vi "MotorUI.vi"() -> ()   [LabVIEW 2011]
uses:
  MotorPosType.ctl
  Typedefs/XYf.ctl
  MotorStateType.ctl
  Typedefs/CmdEnum_MotorIn.ctl
  MotorAxisEnum.ctl
  MotorCmd_MoveToLimit.ctl
  GlobalVariables.vi
panel:
  in  "Cam XY Control":T1
  out "Cam Y":sgl
  out "Cam X":sgl
  in  "Save config":bool
  in  "Piezo XY":T1
  out "Piezo Y":sgl
  out "Piezo X":sgl
  out "Focal depth (um):":sgl
  out "Rotation (turns):":sgl
  out "Position: (mm)":sgl
  out "Motor update lag counter":i32
  in  "Rotation speed\n(turns/s)":sgl=1.0
  in  "Magnet offset":sgl
  in  "Piezo step pageup/down":sgl=2.0
  in  "Magnet home":bool
  in  "Reset magnet zero pos":bool
  out "Offset":T2
  in  "MotorState (initial value)":T3
  in  "Step size of up/down buttons":sgl=3.0
  in  "Motors Initialized?":bool
  out "motor cmd queue len":i32
  out "Current Position":T2
  in  "Piezo position":sgl
  in  "Magnet position [mm]":sgl
  in  "Rotation [turns]":sgl
  in  "Move magnet up":bool
  in  "Move magnet down":bool
  in  "Magnet rotation: Alternate 0/10":bool
  in  "Piezo stage down":bool
  in  "Piezo stage up":bool
  in  "Piezo step:":sgl=5.0
  # "Magnet Z"
  # "Focal depth"
  # "Magnet Rotation"
  # "Piezo XY"
  # "Magnet position:\nThe shown 'magnet position' cannot go below zero, so you can use the offset to set a lower magnet limit (in order to protect your flowcell)"
  # "Camera XY"
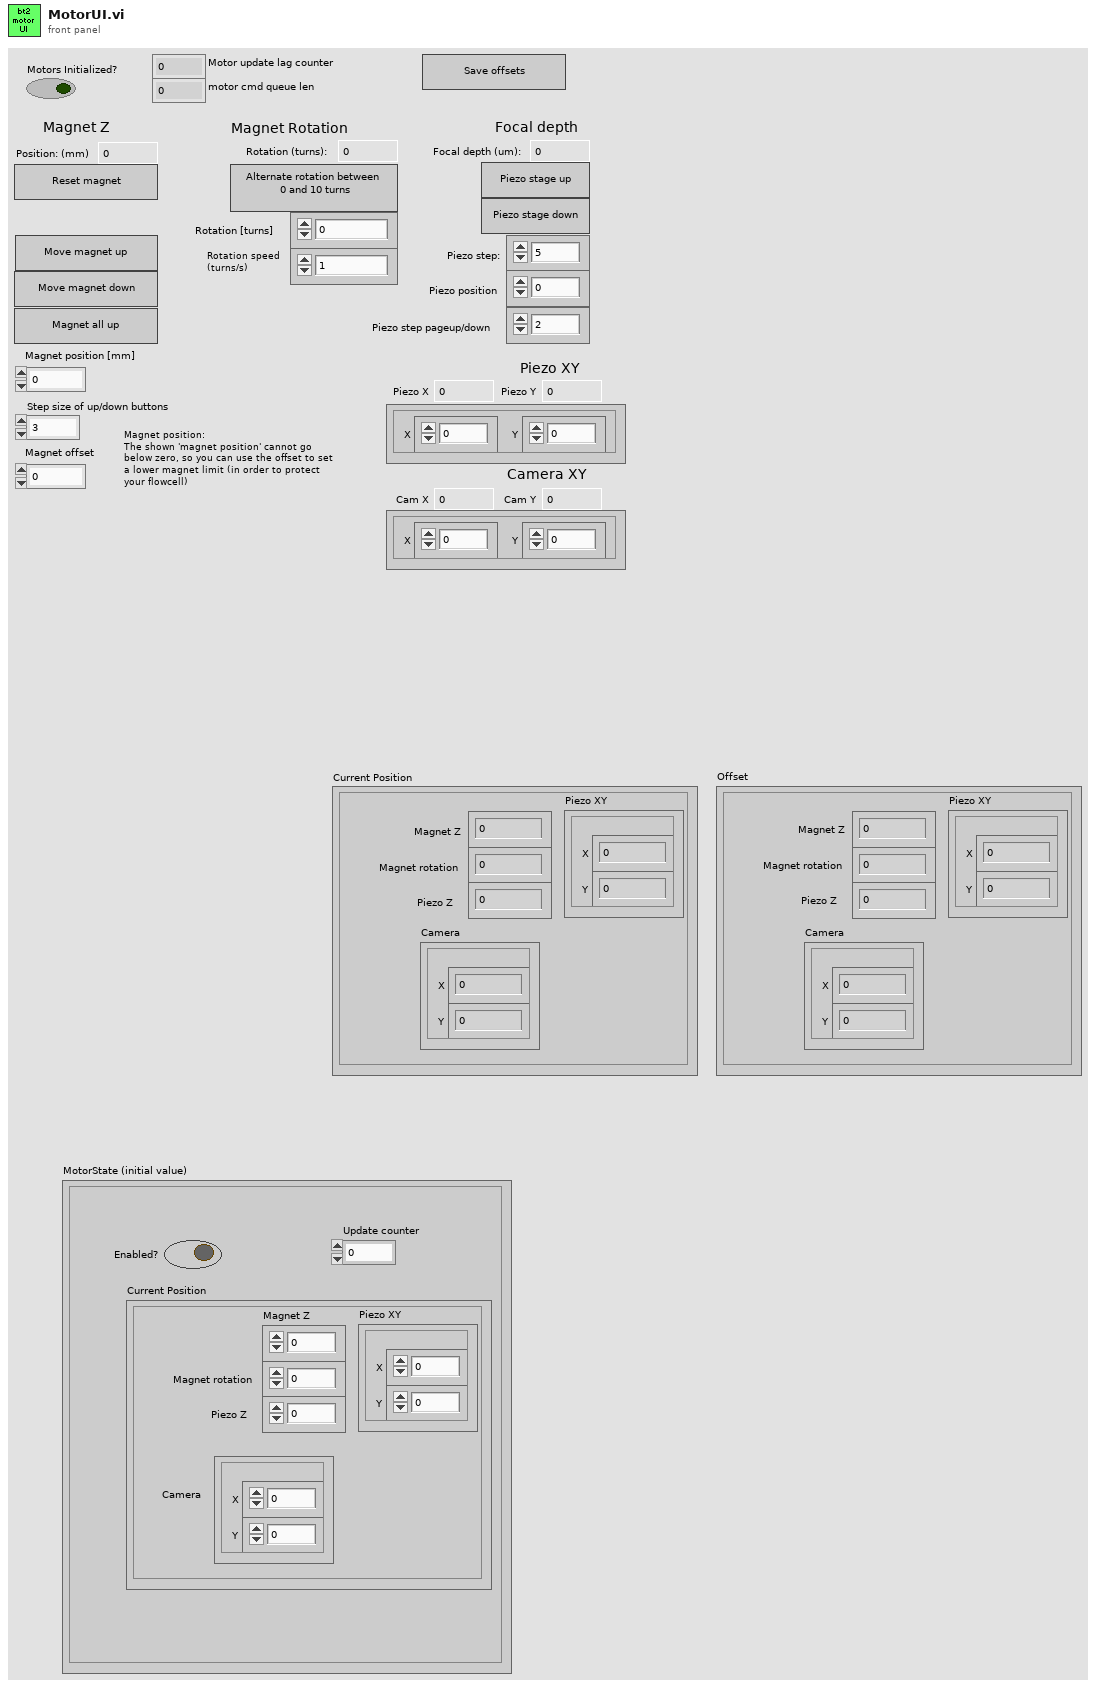
[diagram p1: front panel]
types:
  T1 = typedef "XYf.ctl" = cluster{"X":sgl, "Y":sgl}
  T2 = typedef "MotorPosType.ctl" = cluster{"Magnet Z":dbl, "Magnet rotation":dbl, "Camera":T1, "Piezo XY":T1, "Piezo Z":dbl}
  T3 = typedef "MotorStateType.ctl" = cluster{"Enabled?":bool, "Current Position":T2, "Update counter":i32}
  T4 = typedef "MotorConfigType.ctl" = cluster{"Offset":T2, "Maximum pos":T2, "Min limited?":T5, "Max limited?":T5, "Has velocity support":T5, "Default velocity":T2}
  T5 = typedef "MotorPosFlagsType.ctl" = cluster{"Magnet Z":bool, "Magnet rotation":bool, "Camera":cluster{"X":bool, "Y":bool}, "Piezo XY":cluster{"X":bool, "Y":bool}, "Piezo Z":bool}
  T6 = typedef "MotorAxisEnum.ctl" = enum16{"no axis", "magrot", "magpos", "px", "py", "pz", "camx", "camy"}
  T7 = typedef "CmdEnum_MotorIn.ctl" = enum32{"Init", "Close", "SetPosition", "UpdatePositions", "MoveToLimit"}
  T8 = typedef "MotorCmd_MoveToLimit.ctl" = cluster{"Motor Axis":T6, "Limit switch":enum16{"Positive", "Negative"}}
  T9 = typedef "eventvkey.ctl" = enum16{"ASCII", "Enter", "Return", "Shift", "Ctrl", "Alt", "Cmd", "Opt", "Caps", "NumLock", "Clear", "Break", "Up", "Down", "Left", "Right", "Insert", "Delete", "Home", "End", "PageUp", "PageDown", "Escape", "Help", "Pause", "ScrollLock", "F1", "F2", "F3", "F4", "F5", "F6", "F7", "F8", "F9", "F10", "F11", "F12", "F13", "F14", "F15", "F16", "F17", "F18", "F19", "F20", "F21", "F22", "F23", "F24", "Play", "VolumeUp", "VolumeDown", "Mute", "Two Byte Char"}
  T10 = typedef "QueueListType.ctl" = cluster{"Motor In":refnum<queue>, "User Interface Image View":refnum<queue>, "User Interface Camera Control":refnum<queue>, "User Interface Event Notifier":refnum<notifier>, "Initialized?":bool, "Experiment Script Event Notifier":refnum<notifier>}
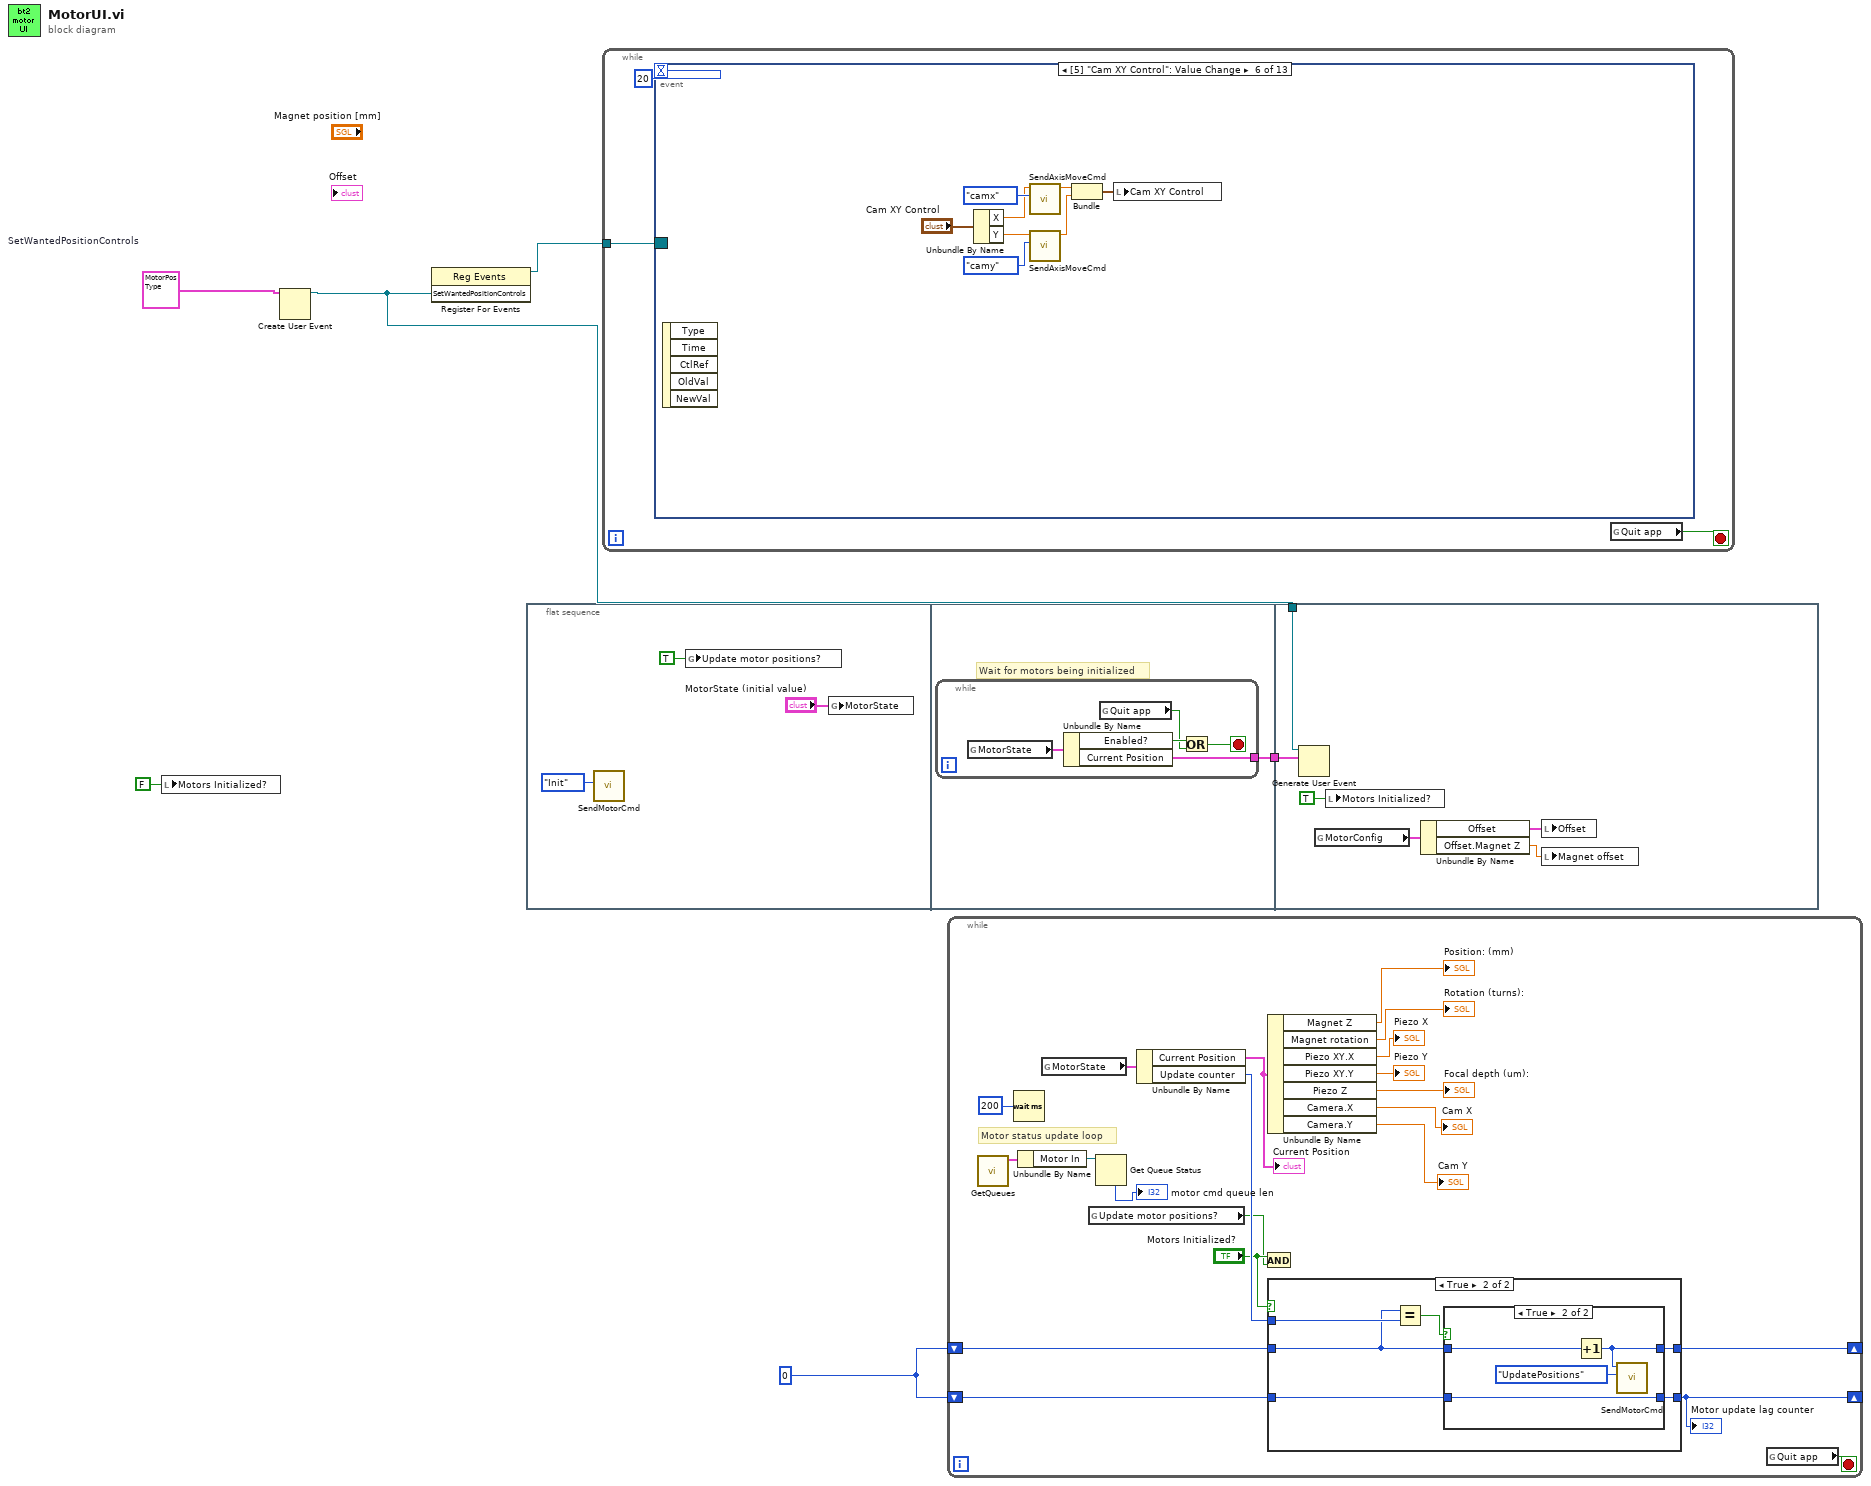
[diagram p0: block diagram]
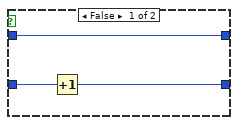
[diagram p3: hidden frame]
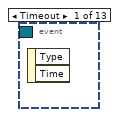
[diagram p4: hidden frame]
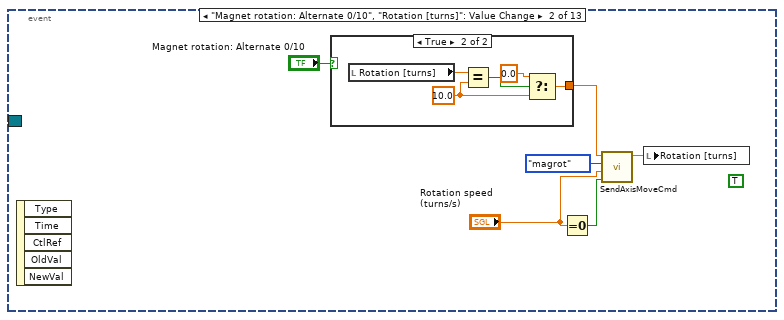
[diagram p5: hidden frame]
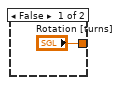
[diagram p6: hidden frame]
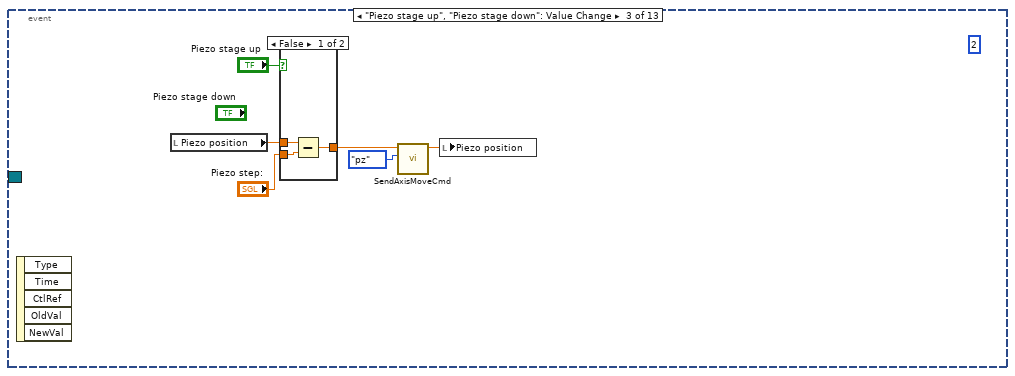
[diagram p7: hidden frame]
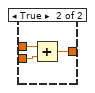
[diagram p8: hidden frame]
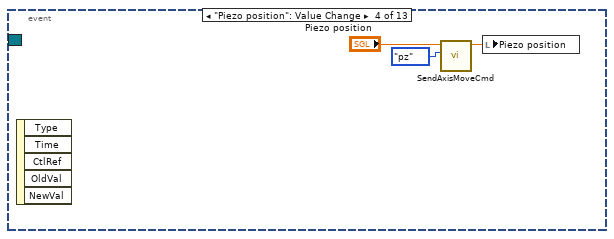
[diagram p9: hidden frame]
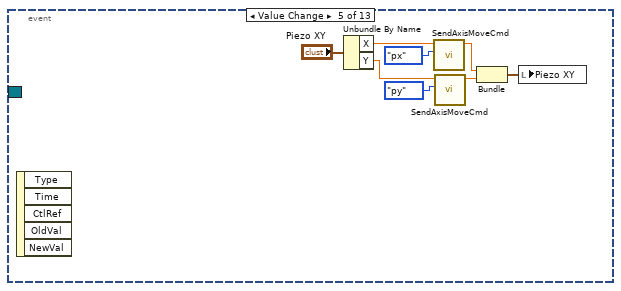
[diagram p10: hidden frame]
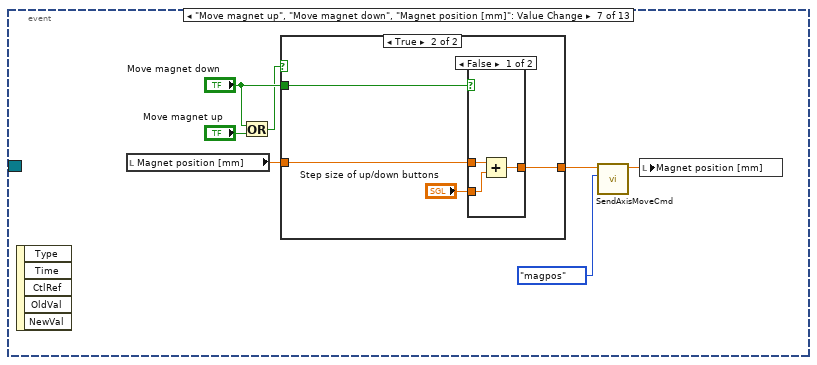
[diagram p11: hidden frame]
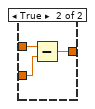
[diagram p13: hidden frame]
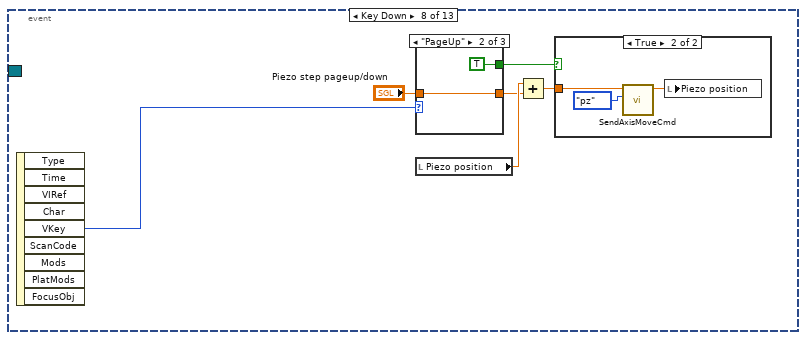
[diagram p14: hidden frame]
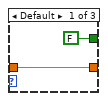
[diagram p16: hidden frame]
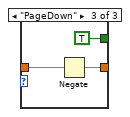
[diagram p17: hidden frame]
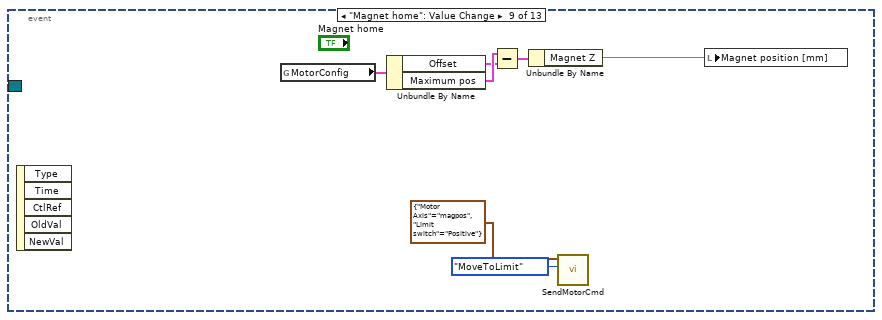
[diagram p18: hidden frame]
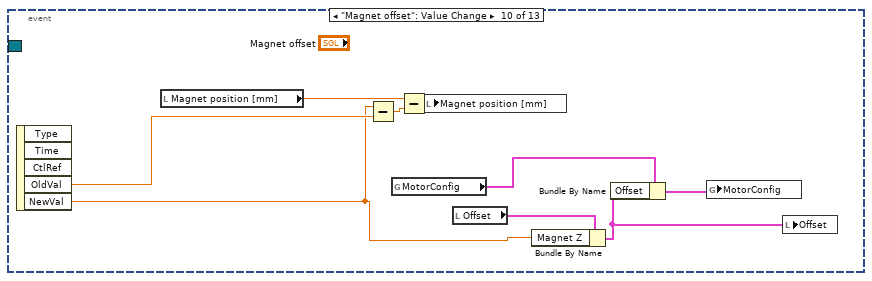
[diagram p19: hidden frame]
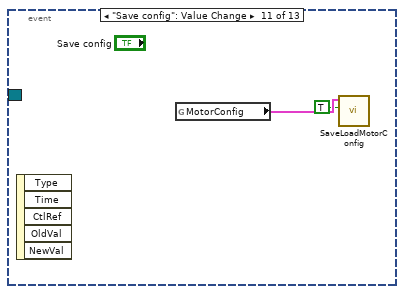
[diagram p20: hidden frame]
diagram:
  w4 = 0 ("Update counter")
  w5 = T2 {"Magnet Z"=0.0, "Magnet rotation"=0.0, "Camera"={"X"=0.0, "Y"=0.0}, "Piezo XY"={"X"=0.0, "Y"=0.0}, "Piezo Z"=0.0}  # SetWantedPositionControls
  n1 = local write "Motors Initialized?"(FALSE ("Motor Initialized?")) -> ()
  n2 = Create User Event(user event datatype=w5) -> (user event=w1:refnum<user-event>)  [unwired: 1 in, 1 out]
  n3 = register-events(w1) -> (reference out=w3:refnum<event-registration>)  [unwired: 2 in, 1 out]
  n4 = flat-sequence {
    tunnel: [w10] -> w2
    tunnel: w1 -> [w20]
    tunnel: w2 -> [w19]
    frame #0 {
      n5 = call "SendMotorCmd.vi"("Command Type"=enum16{"Init", "Close", "SetPosition"}."Init") -> ()  [unwired: 11 in]
      n6 = global write "GlobalVariables.vi" "Update motor positions?"(TRUE ("Update motor positions?")) -> ()
      n7 = global write "GlobalVariables.vi" "MotorState"("MotorState (initial value)") -> ()
    }
    frame #1 {
      # "Wait for motors being initialized"
      n8 = while {
        tunnel: [w14] -> w10
        stop <- w11 stop-if-true
        n9 = global read "GlobalVariables.vi" "MotorState"() -> (w15:T3)
        n10 = Unbundle By Name(w15) -> ("Enabled?"=w13:bool, "Current Position"=w14:T2)
        n11 = global read "GlobalVariables.vi" "Quit app"() -> (w12:bool)
        n12 = Or(x=w13, y=w12) -> (x .or. y?=w11:bool)
      }
    }
    frame #2 {
      n13 = Generate User Event(user event=w20, event data cluster=w19) -> ()  [unwired: 1 in, 2 out]
      n14 = global read "GlobalVariables.vi" "MotorConfig"() -> (w18:T4)
      n15 = local write "Motors Initialized?"(TRUE ("Motor Initialized?")) -> ()
      n16 = Unbundle By Name(w18) -> ("Offset"=w16:T2, "Offset.Magnet Z"=w17:dbl)
      n17 = local write "Offset"(w16) -> ()
      n18 = local write "Magnet offset"(w17) -> ()
    }
  }
  n19 = while {
    tunnel: w3 -> [w22]
    stop <- w23 stop-if-true
    n20 = event shown="[5] \"Cam XY Control\": Value Change" {
      selector: w22 -> [_ _ _ _ _ _ _ _ _ _ _ _ _]
      dyn-events: _ -> [_ _ _ _ _ _ _ _ _ _ _ _ _]
      timeout: 20 -> [_ _ _ _ _ _ _ _ _ _ _ _ _]
      event Timeout {
        n21 = event-data() -> ()  [unwired: 1 in, 2 out]
      }
      event "Magnet rotation: Alternate 0/10", "Rotation [turns]": Value Change {
        (unwired) TRUE ("Move flags.Magnet rotation")
        n22 = event-data() -> ()  [unwired: 1 in, 5 out]
        n23 = case shown="True" "Magnet rotation: Alternate 0/10" {
          tunnel: ["Rotation [turns]" w32] -> w28
          frame False {
          }
          frame True {
            w33 = sgl 10.0 ("y")
            n24 = local read "Rotation [turns]"() -> (w36:sgl)
            n25 = Equal?(x=w36, y=w33) -> (x = y?=w35:bool)
            n26 = Select(t=0.0, s=w35, f=w33) -> (s? t:f=w32:dbl)
          }
        }
        n27 = Equal To 0?(x="Rotation speed\n(turns/s)") -> (x = 0?=w25:bool)
        n28 = call "SendAxisMoveCmd.vi"("Instant? (T)"=w25, "Speed"="Rotation speed\n(turns/s)", "axis"=MotorAxisEnum."magrot", "Position"=w28) -> ("Limited pos"=w29:dbl)  [unwired: 7 in]
        n29 = local write "Rotation [turns]"(w29) -> ()
      }
      event "Piezo stage up", "Piezo stage down": Value Change {
        (unwired) 2 ("axis index")
        n30 = event-data() -> ()  [unwired: 1 in, 5 out]
        n31 = local read "Piezo position"() -> (w40:sgl)
        n32 = case shown="False" "Piezo stage up" {
          tunnel: w40 -> [w45 w48]
          tunnel: "Piezo step:" -> [w44 w47]
          tunnel: [w43 w46] -> w38
          frame False {
            n33 = Subtract(x=w45, y=w44) -> (x-y=w43:sgl)
          }
          frame True {
            n34 = Add(x=w48, y=w47) -> (x+y=w46:sgl)
          }
        }
        n35 = call "SendAxisMoveCmd.vi"("axis"=MotorAxisEnum."pz", "Position"=w38) -> ("Limited pos"=w39:dbl)  [unwired: 9 in]
        n36 = local write "Piezo position"(w39) -> ()
      }
      event "Piezo position": Value Change {
        n37 = event-data() -> ()  [unwired: 1 in, 5 out]
        n38 = call "SendAxisMoveCmd.vi"("axis"=MotorAxisEnum."pz", "Position"="Piezo position") -> ("Limited pos"=w49:dbl)  [unwired: 9 in]
        n39 = local write "Piezo position"(w49) -> ()
      }
      event Value Change {
        n40 = event-data() -> ()  [unwired: 1 in, 5 out]
        n41 = Unbundle By Name("Piezo XY") -> ("X"=w58:sgl, "Y"=w57:sgl)
        n42 = call "SendAxisMoveCmd.vi"("axis"=MotorAxisEnum."px", "Position"=w58) -> ("Limited pos"=w54:dbl)  [unwired: 9 in]
        n43 = call "SendAxisMoveCmd.vi"("axis"=MotorAxisEnum."py", "Position"=w57) -> ("Limited pos"=w53:dbl)  [unwired: 9 in]
        n44 = Bundle("Limited pos"=w54, "Limited pos"=w53) -> (w52:cluster{"Limited pos":dbl, "Limited pos":dbl})  [unwired: 1 in]
        n45 = local write "Piezo XY"(w52) -> ()
      }
      event Value Change {
        n46 = event-data() -> ()  [unwired: 1 in, 5 out]
        n47 = Unbundle By Name("Cam XY Control") -> ("X"=w62:sgl, "Y"=w61:sgl)
        n48 = call "SendAxisMoveCmd.vi"("axis"=MotorAxisEnum."camx", "Position"=w62) -> ("Limited pos"=w65:dbl)  [unwired: 9 in]
        n49 = call "SendAxisMoveCmd.vi"("axis"=MotorAxisEnum."camy", "Position"=w61) -> ("Limited pos"=w64:dbl)  [unwired: 9 in]
        n50 = Bundle("Limited pos"=w65, "Limited pos"=w64) -> (w60:cluster{"Limited pos":dbl, "Limited pos":dbl})  [unwired: 1 in]
        n51 = local write "Cam XY Control"(w60) -> ()
      }
      event "Move magnet up", "Move magnet down", "Magnet position [mm]": Value Change {
        n52 = event-data() -> ()  [unwired: 1 in, 5 out]
        n53 = local read "Magnet position [mm]"() -> (w71:sgl)
        n54 = Or(x="Move magnet down", y="Move magnet up") -> (x .or. y?=w72:bool)
        n55 = case shown="True" w72 {
          tunnel: w71 -> [w75 w79]
          tunnel: "Move magnet down" -> [_ w77]
          tunnel: [w75 w76] -> w69
          frame False {
          }
          frame True {
            n56 = case shown="False" w77 {
              tunnel: w79 -> [w82 w85]
              tunnel: "Step size of up/down buttons" -> [w81 w84]
              tunnel: [w80 w83] -> w76
              frame False {
                n57 = Add(x=w82, y=w81) -> (x+y=w80:sgl)
              }
              frame True {
                n58 = Subtract(x=w85, y=w84) -> (x-y=w83:sgl)
              }
            }
          }
        }
        n59 = call "SendAxisMoveCmd.vi"("axis"=MotorAxisEnum."magpos", "Position"=w69) -> ("Limited pos"=w68:dbl)  [unwired: 9 in]
        n60 = local write "Magnet position [mm]"(w68) -> ()
      }
      event Key Down {
        n61 = event-data() -> ("VKey"=w91:T9)  [unwired: 1 in, 8 out]
        n62 = case shown="\"PageUp\"" w91 {
          tunnel: [FALSE TRUE TRUE] -> w90
          tunnel: "Piezo step pageup/down" -> [w95 w97 w100]
          tunnel: [w95 w97 w99] -> w87
          frame Default {
          }
          frame "PageUp" {
          }
          frame "PageDown" {
            n63 = Negate(x=w100) -> (-x=w99:sgl)
          }
        }
        n64 = local read "Piezo position"() -> (w88:sgl)
        n65 = Add(x=w88, y=w87) -> (x+y=w86:sgl)
        n66 = case shown="True" w90 {
          tunnel: w86 -> [_ w93]
          frame False {
          }
          frame True {
            n67 = call "SendAxisMoveCmd.vi"("axis"=MotorAxisEnum."pz", "Position"=w93) -> ("Limited pos"=w92:dbl)  [unwired: 9 in]
            n68 = local write "Piezo position"(w92) -> ()
          }
        }
      }
      event "Magnet home": Value Change {
        n69 = event-data() -> ()  [unwired: 1 in, 5 out]
        n70 = global read "GlobalVariables.vi" "MotorConfig"() -> (w108:T4)
        n71 = Unbundle By Name(w108) -> ("Offset"=w106:T2, "Maximum pos"=w107:T2)
        n72 = Subtract(x=w107, y=w106) -> (x-y=w105:T2)
        n73 = Unbundle By Name(w105) -> ("Magnet Z"=w102:dbl)
        n74 = call "SendMotorCmd.vi"("Command Type"=CmdEnum_MotorIn."MoveToLimit", "Command Data"=T8 {"Motor Axis"=enum."magpos", "Limit switch"=enum."Positive"} ("MotorCmd_MoveToLimit")) -> ()  [unwired: 10 in]
        n75 = local write "Magnet position [mm]"(w102) -> ()
      }
      event "Magnet offset": Value Change {
        n76 = event-data() -> ("OldVal"=w117:sgl, "NewVal"=w110:sgl)  [unwired: 1 in, 3 out]
        n77 = local read "Magnet position [mm]"() -> (w116:sgl)
        n78 = Subtract(x=w110, y=w117) -> (x-y=w115:sgl)
        n79 = global read "GlobalVariables.vi" "MotorConfig"() -> (w113:T4)
        n80 = Subtract(x=w116, y=w115) -> (x-y=w114:sgl)
        n81 = local write "Magnet position [mm]"(w114) -> ()
        n82 = local read "Offset"() -> (w111:T2)
        n83 = Bundle By Name(cluster=w111, "Magnet Z"=w110) -> (w109:T2)
        n84 = Bundle By Name(cluster=w113, "Offset"=w109) -> (w112:T4)
        n85 = global write "GlobalVariables.vi" "MotorConfig"(w112) -> ()
        n86 = local write "Offset"(w109) -> ()
      }
      event "Save config": Value Change {
        n87 = event-data() -> ()  [unwired: 1 in, 5 out]
        n88 = global read "GlobalVariables.vi" "MotorConfig"() -> (w119:T4)
        n89 = call "SaveLoadMotorConfig.vi"("Save? (F)"=TRUE ("Save?"), "MotorConfig(in)"=w119) -> ()  [unwired: 7 in, 3 out]
      }
      event "Reset magnet zero pos": Value Change {
        n90 = event-data() -> ()  [unwired: 1 in, 5 out]
        n91 = flat-sequence {
          tunnel: [w126] -> w122
          tunnel: [w124] -> w121
          tunnel: [w123] -> w120
          tunnel: w122 -> [w132]
          tunnel: w121 -> [w130]
          tunnel: w120 -> [w129]
          frame #0 {
            n92 = global read "GlobalVariables.vi" "MotorConfig"() -> (w127:T4)
            n93 = Bundle By Name(cluster=w127, "Offset.Magnet Z"=0.0) -> (w125:T4)
            n94 = Unbundle By Name(w127) -> ("Offset.Magnet Z"=w126:dbl)
            n95 = global write "GlobalVariables.vi" "MotorConfig"(w125) -> ()
            n96 = Unbundle By Name(w125) -> ("Offset"=w124:T2, "Offset.Magnet Z"=w123:dbl)
          }
          frame #1 {
            n97 = local read "Magnet position [mm]"() -> (w133:sgl)
            n98 = local write "Magnet offset"(w129) -> ()
            n99 = Add(x=w132, y=w133) -> (x+y=w131:dbl)
            n100 = local write "Magnet position [mm]"(w131) -> ()
            n101 = local write "Offset"(w130) -> ()
          }
        }
      }
      event User Event {
        n102 = event-data() -> ("Magnet Z"=w137:dbl, "Magnet rotation"=w136:dbl, "Piezo XY"=w134:T1, "Piezo Z"=w135:dbl)  [unwired: 1 in, 4 out]
        n103 = local write "Piezo position"(w135) -> ()
        n104 = local write "Magnet position [mm]"(w137) -> ()
        n105 = local write "Rotation [turns]"(w136) -> ()
        n106 = local write "Piezo XY"(w134) -> ()
      }
    }
    n107 = global read "GlobalVariables.vi" "Quit app"() -> (w23:bool)
  }
  n108 = while {
    shift-right: [w150] -> _
    shift-left: w4 -> [w151]
    shift-right: [w148] -> _
    shift-left: w4 -> [w149]
    stop <- w157 stop-if-true
    # "Motor status update loop"
    n109 = call "GetQueues.vi"() -> ("Queue List"=w155:T10)  [unwired: 10 in, 1 out]
    n110 = Wait (ms)(milliseconds to wait=u32 200) -> ()  [unwired: 1 out]
    n111 = Unbundle By Name(w155) -> ("Motor In"=w154:refnum<queue>)
    n112 = global read "GlobalVariables.vi" "MotorState"() -> (w156:T3)
    n113 = global read "GlobalVariables.vi" "Update motor positions?"() -> (w146:bool)
    n114 = Get Queue Status(queue=w154) -> (# elements in queue=→"motor cmd queue len":i32)  [unwired: 2 in, 7 out]
    n115 = Unbundle By Name(w156) -> ("Current Position"=w145:T2, "Update counter"=w152:i32)
    "Current Position" <- w145
    n116 = And(x="Motors Initialized?", y=w146) -> ()  [unwired: 1 out]
    n117 = Unbundle By Name(w145) -> ("Magnet Z"=→"Position: (mm)":dbl, "Magnet rotation"=→"Rotation (turns):":dbl, "Piezo XY.X"=→"Piezo X":sgl, "Piezo XY.Y"=→"Piezo Y":sgl, "Piezo Z"=→"Focal depth (um):":dbl, "Camera.X"=→"Cam X":sgl, "Camera.Y"=→"Cam Y":sgl)
    n118 = case shown="True" "Motors Initialized?" {
      tunnel: w152 -> [_ w166]
      tunnel: w151 -> [w160 w162]
      tunnel: [w160 w161] -> w150
      tunnel: w149 -> [w159 w164]
      tunnel: [w159 w163] -> w148
      frame False {
      }
      frame True {
        n119 = Equal?(x=w162, y=w166) -> (x = y?=w165:bool)
        n120 = case shown="True" w165 {
          tunnel: w162 -> [w167 w171]
          tunnel: w164 -> [w169 w172]
          tunnel: [w168 w172] -> w163
          tunnel: [w167 w170] -> w161
          frame False {
            n121 = Increment(x=w169) -> (x+1=w168:i32)
          }
          frame True {
            n122 = Increment(x=w171) -> (x+1=w170:i32)
            n123 = call "SendMotorCmd.vi"("Command Type"=CmdEnum_MotorIn."UpdatePositions", "Command Data"=w170) -> ()  [unwired: 10 in]
          }
        }
      }
    }
    "Motor update lag counter" <- w148
    n124 = global read "GlobalVariables.vi" "Quit app"() -> (w157:bool)
  }
